vi "Set channel.vi"(8 "error in (no error)":errorcluster, 10 "channel":i32=36, 11 "niDTS WLAN Dut in":refnum<class "niDTS WLAN Dut.lvclass">) -> (0 "error out":errorcluster, 3 "niDTS WLAN Dut out":refnum<class "niDTS WLAN Dut.lvclass">)   [LabVIEW 2015, in "niDTS WLAN.lvlib" / "niDTS WLAN Dut.lvclass"]
uses:
  niDTS WLAN Dut.lvclass
  niDTS WLAN Dut.lvclass/niDTS WLAN Dut.ctl
  niDTS WLAN.lvlib
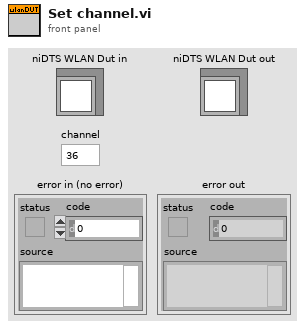
[diagram p1: front panel]
types:
  T1 = typedef "niDTS WLAN.lvlib/niDTS WLAN INC CH BW.ctl" = enum16{"20 MHz", "40 MHz", "80 MHz", "160 MHz"}
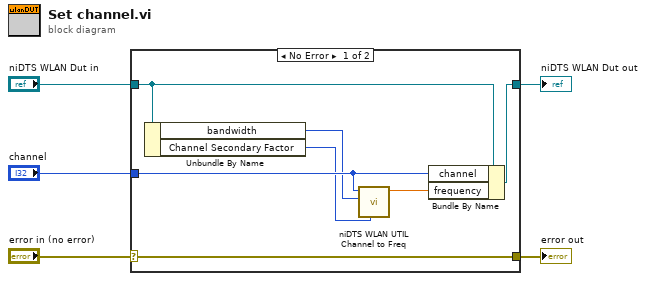
[diagram p0: block diagram]
diagram:
  n1 = case shown="No Error" "error in (no error)" {
    selector: "error in (no error)" -> [w12 w13]
    tunnel: [w12 w13] -> w4
    tunnel: [w11 w14] -> w2
    tunnel: "niDTS WLAN Dut in" -> [w9 w14]
    tunnel: "channel" -> [w10 _]
    frame No Error {
      n2 = Unbundle By Name(w9) -> ("bandwidth"=w8:T1, "Channel Secondary Factor"=w7:i8)
      n3 = call "niDTS WLAN UTIL Channel to Freq.vi"("secondary factor"=w7, "CH BW"=w8, "Channel"=w10) -> ("Center Frequency (Hz)"=w6:dbl)  [unwired: 6 in, 2 out]
      n4 = Bundle By Name(cluster=w9, "channel"=w10, "frequency"=w6) -> (w11:refnum<class "niDTS WLAN Dut.lvclass">)
    }
    frame Error {
    }
  }
  "error out" <- w4
  "niDTS WLAN Dut out" <- w2
